vi "Cargo Intake.vi"   [LabVIEW 2018]
uses:
  <vilib>/Rock Robotics/WPI/Solenoid/WPI_SolenoidChannel.ctl
  <vilib>/Rock Robotics/SystemInterfaces/DIO/FPGA_DIOChannel.ctl
  <vilib>/Rock Robotics/WPI/ThirdParty/Phoenix-LabVIEW/Motor Controller/Controls/CTRE_Phoenix_MotorControl_ControlMode.ctl
  <vilib>/Rock Robotics/WPI/Solenoid/WPI_SolenoidValue.ctl
  <vilib>/Rock Robotics/WPI/Solenoid/WPI_SolenoidOpenSingle.vi
  Times/Times Global.vi
  Cargo Intake Global.vi
  <vilib>/Rock Robotics/WPI/Solenoid/WPI_SolenoidSetEnum.vi
types:
  T1 = typedef "FPGA_DIOChannel.ctl" = enum8{"DIO 0", "DIO 1", "DIO 2", "DIO 3", "DIO 4", "DIO 5", "DIO 6", "DIO 7", "DIO 8", "DIO 9", "DIO MXP 0", "DIO MXP 1", "DIO MXP 2", "DIO MXP 3", "DIO MXP 4", "DIO MXP 5", "DIO MXP 6", "DIO MXP 7", "DIO MXP 8", "DIO MXP 9", "DIO MXP 10", "DIO MXP 11", "DIO MXP 12", "DIO MXP 13", "DIO MXP 14", "DIO MXP 15", "SPI Port CS1", "SPI Port CS2", "SPI Port CS3", "SPI Port MISO", "SPI Port MOSI", "Invalid"}
  T2 = typedef "WPI_SolenoidChannel.ctl" = enum8{"Solenoid 0", "Solenoid 1", "Solenoid 2", "Solenoid 3", "Solenoid 4", "Solenoid 5", "Solenoid 6", "Solenoid 7", "Invalid"}
  T3 = typedef "WPI_SolenoidDevRef.ctl" = cluster{"DevStatus":errorcluster, "Pneumatics Control Module":u8, "Forward Solenoid Channel":T2, "Reverse Solenoid Channel":T2}
  T4 = typedef "WPI_DigitalInputDevRef.ctl" = cluster{"DevStatus":errorcluster, "DIO Channel":T1}
  T5 = typedef "WPI_MotorControlDeviceRef.ctl" = cluster{"DeviceStatus":errorcluster, "Type":T6, "PWM":cluster{"PWM Channel":T7, "DeadBand":T8}, "CAN":cluster{"Device Number":u8, "SetOutput VI Ref":variant, "GetOutput VI Ref":variant, "Enable VI Ref":variant, "Disable VI Ref":variant, "Data":variant}, "Invert":bool, "DIO PWM":cluster{"PWM \"Enable\" Channel":T7, "DIOChannel":T1, "PWM Rate":dbl}}
  T6 = typedef "WPI_MotorControlType.ctl" = enum16{"PWM", "CAN", "DIO PWM"}
  T7 = typedef "FPGA_DIOPWMChannel.ctl" = enum8{"PWM 0", "PWM 1", "PWM 2", "PWM 3", "PWM 4", "PWM 5", "PWM 6", "PWM 7", "PWM 8", "PWM 9", "PWM MXP 0", "PWM MXP 1", "PWM MXP 2", "PWM MXP 3", "PWM MXP 4", "PWM MXP 5", "PWM MXP 6", "PWM MXP 7", "PWM MXP 8", "PWM MXP 9", "Invalid"}
  T8 = typedef "WPI_PWMDeadband.ctl" = cluster{"Name":string, "maxPositivePwm":i32, "minPositivePwm":i32, "centerPwm":i32, "maxNegativePwm":i32, "minNegativePwm":i32, "angularRange":u16}
  T9 = typedef "WPI_SolenoidValue.ctl" = enum16{"Off", "On", "Forward", "Reverse"}
  T10 = typedef "CTRE_Phoenix_MotorControl_ControlMode.ctl" = u16
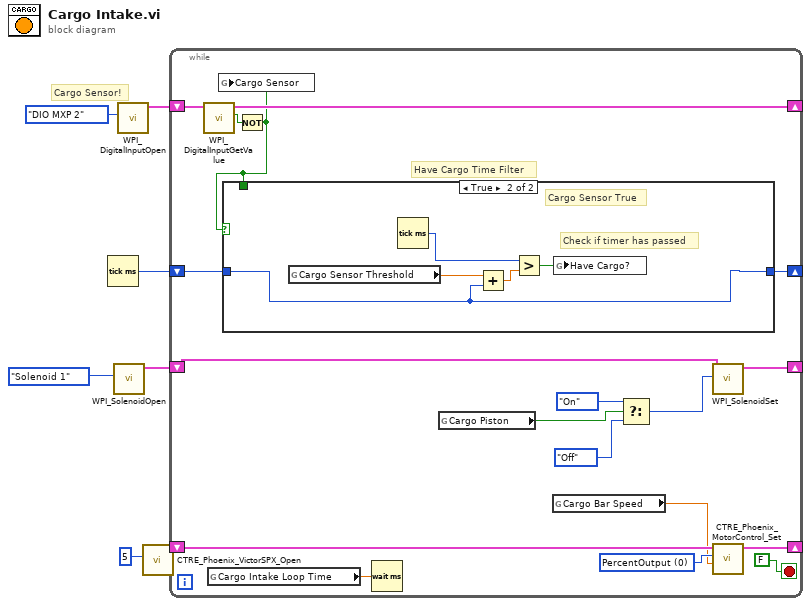
[diagram p0: block diagram]
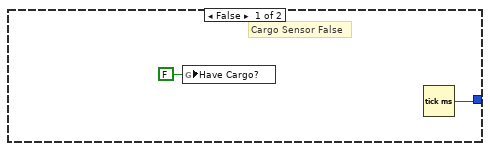
[diagram p2: hidden frame]
diagram:
  # "Cargo Sensor!"
  n1 = Tick Count (ms)() -> (millisecond timer value=w1:u32)
  n2 = call-poly <vilib>:"WPI_SolenoidOpen.vi"("Solenoid Channel"=WPI_SolenoidChannel."Solenoid 1") -> ("SolenoidDevRef"=w4:T3)  [unwired: 9 in, 1 out]
  n3 = call <vilib>:"WPI_DigitalInputOpen.vi"("DIO Channel"=FPGA_DIOChannel."DIO MXP 2") -> ("DigitalInputDevRef"=w3:T4)  [unwired: 9 in, 1 out]
  n4 = call <vilib>:"CTRE_Phoenix_VictorSPX_Open.vi"("Device Number"=u8 5) -> ("CAN Talon SRX Ref"=w6:T5)  [unwired: 9 in, 1 out]
  n5 = while {
    shift-right: [w23] -> _
    shift-left: w6 -> [w21]
    shift-right: [w19] -> _
    shift-left: w4 -> [w17]
    shift-right: [w15] -> _
    shift-left: w3 -> [w16]
    shift-right: [w13] -> _
    shift-left: w1 -> [w14]
    stop <- FALSE stop-if-true
    w22 = T10 0 items=["PercentOutput"=0, "Position"=1, "Velocity"=2, "Current"=3, "Follower"=5, "MotionProfile"=6, "MotionMagic"=7, "MotionProfileArc"=10, "Disabled"=15] ("Control Mode")
    # "Have Cargo Time Filter"
    n6 = call <vilib>:"WPI_DigitalInputGetValue.vi"("DigitalInputDevRef"=w16) -> ("Value"=w12:bool, "DigitalInputDevRef"=w15:T4)  [unwired: 8 in, 1 out]
    n7 = global read "Times Global.vi" "Cargo Intake Loop Time"() -> (w25:dbl)
    n8 = Not(x=w12) -> (.not. x?=w11:bool)
    n9 = global write "Cargo Intake Global.vi" "Cargo Sensor"(w11) -> ()
    n10 = case shown="True" w11 {
      tunnel: w14 -> [_ w29]
      tunnel: [w26 w29] -> w13
      tunnel: w11 -> [_ _]
      frame False {
        # "Cargo Sensor False"
        n11 = global write "Cargo Intake Global.vi" "Have Cargo?"(FALSE ("Have Cargo?")) -> ()
        n12 = Tick Count (ms)() -> (millisecond timer value=w26:u32)
      }
      frame True {
        # "Check if timer has passed"
        # "Cargo Sensor True"
        n13 = global read "Cargo Intake Global.vi" "Cargo Sensor Threshold"() -> (w28:dbl)
        n14 = Tick Count (ms)() -> (millisecond timer value=w31:u32)
        n15 = Add(x=w28, y=w29) -> (x+y=w30:dbl)
        n16 = Greater?(x=w31, y=w30) -> (0:w32:bool)
        n17 = global write "Cargo Intake Global.vi" "Have Cargo?"(w32) -> ()
      }
    }
    n18 = Wait (ms)(milliseconds to wait=w25) -> ()  [unwired: 1 out]
    n19 = global read "Cargo Intake Global.vi" "Cargo Piston"() -> (w8:bool)
    n20 = global read "Cargo Intake Global.vi" "Cargo Bar Speed"() -> (w20:dbl)
    n21 = Select(t=WPI_SolenoidValue."On" ("Value"), s=w8, f=WPI_SolenoidValue."Off" ("Value")) -> (s? t:f=w18:T9)
    n22 = call-poly <vilib>:"WPI_SolenoidSet.vi"("Value"=w18, "SolenoidDevRef"=w17) -> ("SolenoidDevRef"=w19:T3)  [unwired: 8 in, 1 out]
    n23 = call <vilib>:"CTRE_Phoenix_MotorControl_Set.vi"("Output"=w20, "Control Mode"=w22, "PhoenixMotorControlDevRef"=w21) -> ("PhoenixMotorControlDevRef"=w23:T5)  [unwired: 7 in, 1 out]
  }
